vi "SpinnyDebugger.vi"() -> ()   [LabVIEW 2014]
uses:
  <vilib>/userdefined/High Color/IMAQdx.ctl
  <vilib>/LabVIEW Interface for Arduino/LabVIEW Interface for Arduino.lvlib
  <vilib>/vision/driver/NI_Vision_Acquisition_Software.lvlib
  <resource>/objmgr/imaqdx.rc
panel:
  in  "Exposure":u32=3000
  in  "Camera":T1
  out "Image":T2(plugin-control)
  in  "Angular Increment":dbl=5.0
  in  "Captured Image Folder":path
  in  "Camera Mode":enum32{"None", "Triggered", "Live"}(radio)
  in  "Direction":bool=TRUE
  in  "Exit":bool
  in  "home":bool
  in  "stop":bool
  in  "MoveToGo":bool
  in  "Move To":sgl min=0 max=360
  in  "MoveForGo":bool
  in  "Move For (+/-360 max)":sgl=360.0 min=0 max=360
  out "Current Position":sgl format="%.2f"
  # "CW"
  # "CCW"
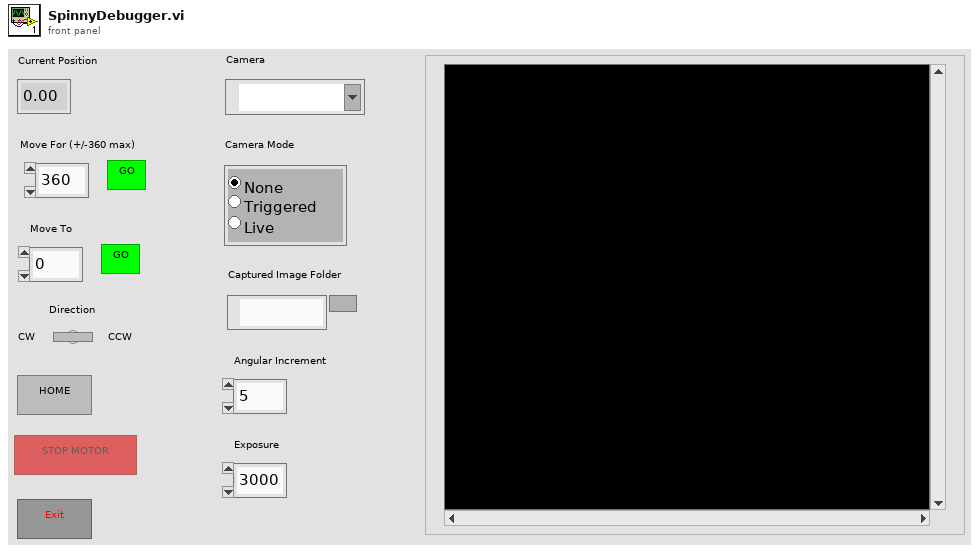
[diagram p1: front panel]
types:
  T1 = typedef "IMAQdx.ctl" = refnum<k21>
  T2 = typedef "IMAQ Image.ctl" = refnum<image>
  T3 = enum8{"Enabled", "Disabled", "Disabled and Grayed Out"}
  T4 = typedef "LabVIEW Interface for Arduino.lvlib/Arduino Resource.ctl" = cluster{"VISA resource":refnum<visa-resource-name>, "Board Type":T5, "Connection Type":enum8{"USB / Serial"}, "Bytes Per Packet (15)":u8}
  T5 = typedef "LabVIEW Interface for Arduino.lvlib/Board Type.ctl" = enum16{"Uno", "Dimuelanove w/Atmega 328", "Mega 2560"}
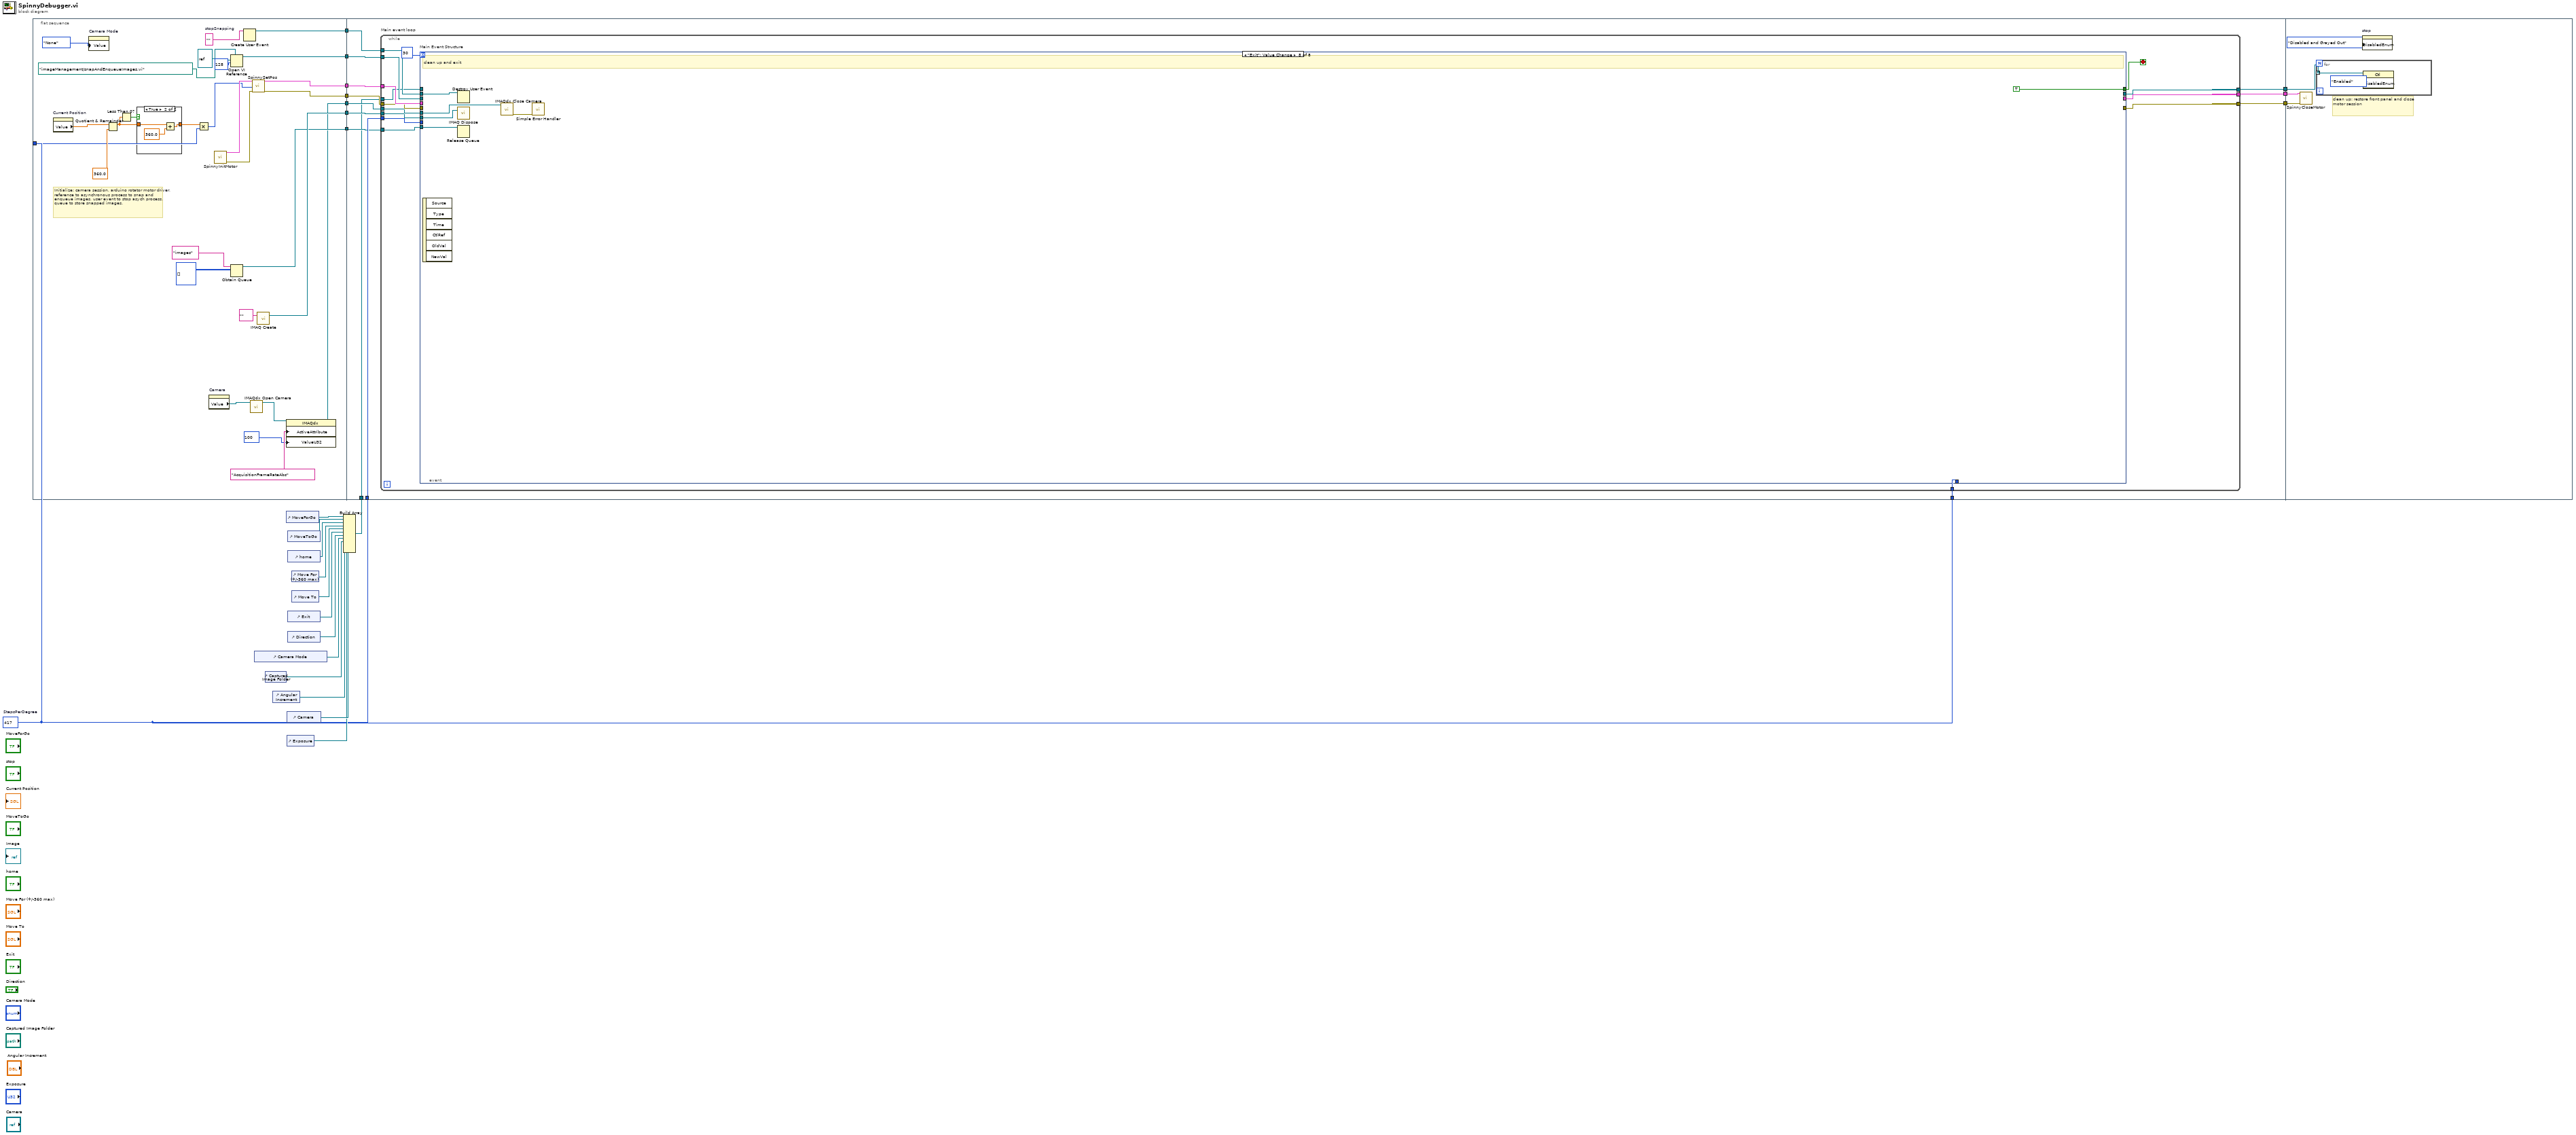
[diagram p0: block diagram]
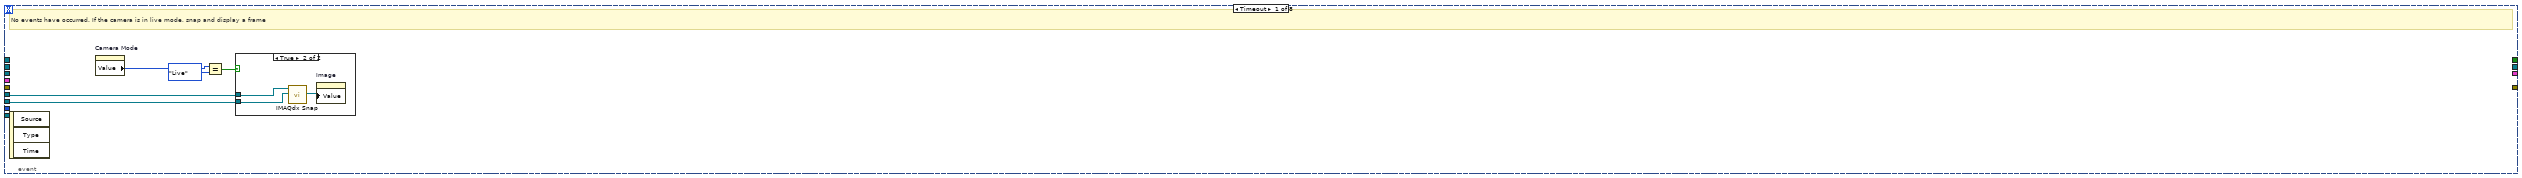
[diagram p3: hidden frame]
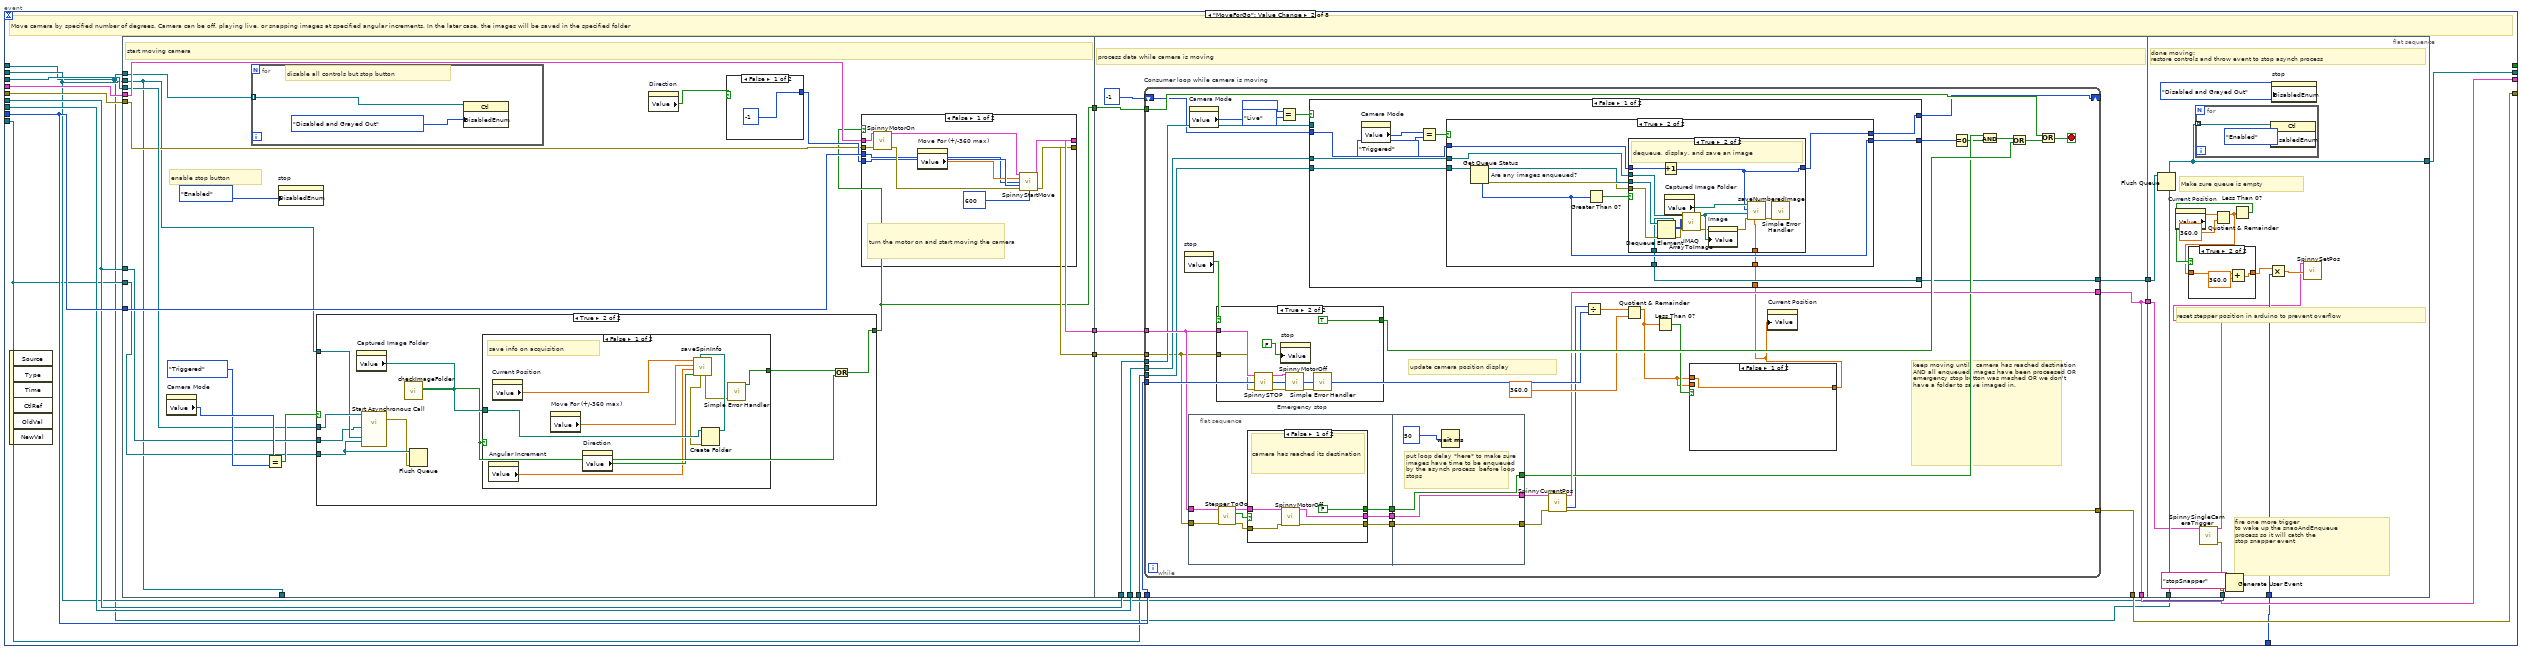
[diagram p5: hidden frame]
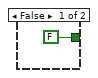
[diagram p7: hidden frame]
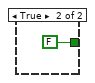
[diagram p8: hidden frame]
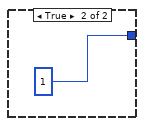
[diagram p9: hidden frame]
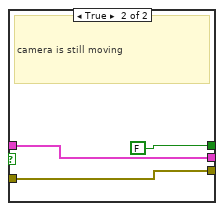
[diagram p10: hidden frame]
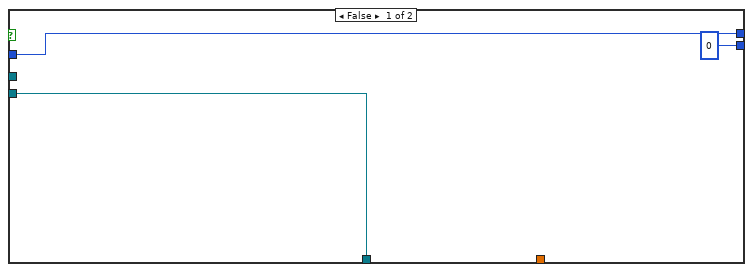
[diagram p11: hidden frame]
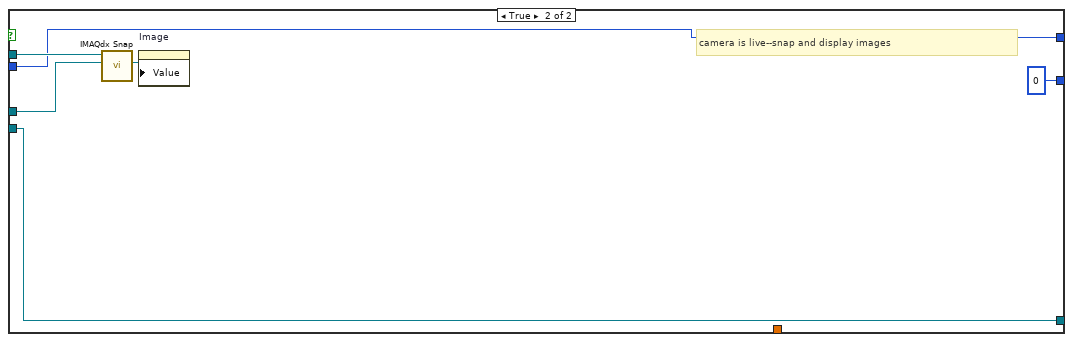
[diagram p13: hidden frame]
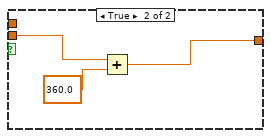
[diagram p14: hidden frame]
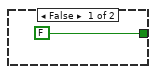
[diagram p15: hidden frame]
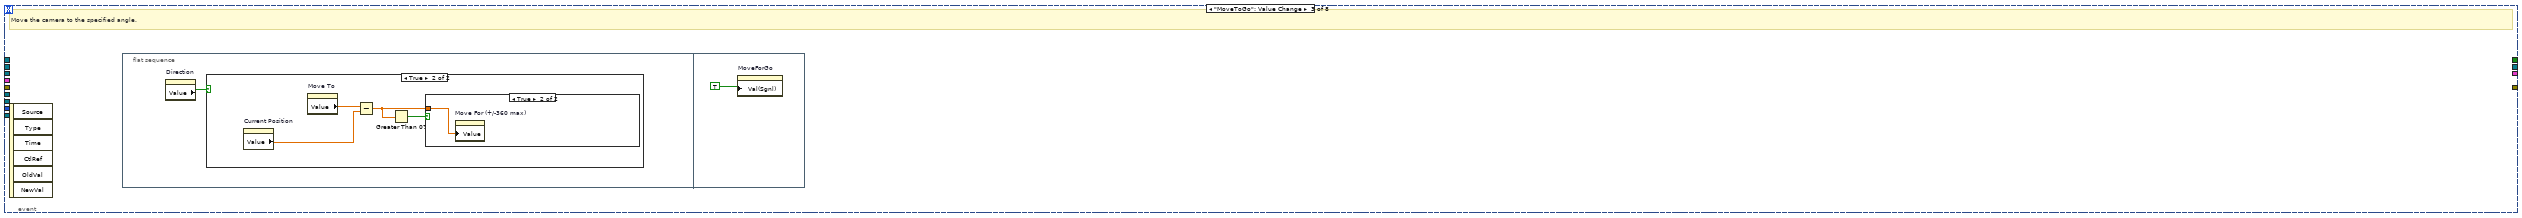
[diagram p17: hidden frame]
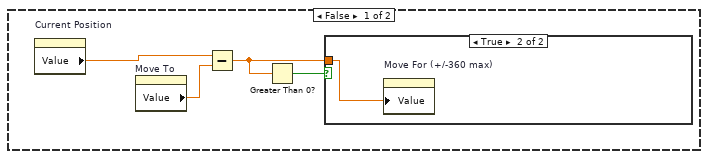
[diagram p18: hidden frame]
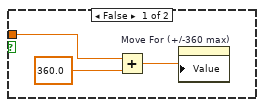
[diagram p19: hidden frame]
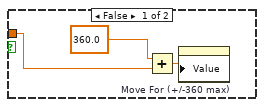
[diagram p20: hidden frame]
diagram:
  w1 = 417  # StepsPerDegree
  n1 = flat-sequence {
    tunnel: [w50] -> w24
    tunnel: [w49] -> w23
    tunnel: w1 -> [w43]
    tunnel: [w27] -> w20
    tunnel: [w39] -> w19
    tunnel: [w33] -> w18
    tunnel: [w31] -> w17
    tunnel: [w30] -> w16
    tunnel: w24 -> [w69]
    tunnel: w23 -> [w68]
    tunnel: w1 -> [w67]
    tunnel: [w66] -> w22
    tunnel: [w65] -> w21
    tunnel: w20 -> [w64]
    tunnel: w19 -> [w63]
    tunnel: w18 -> [w62]
    tunnel: w17 -> [w61]
    tunnel: w16 -> [w60]
    tunnel: w4 -> [w59]
    tunnel: [w58] -> w3
    tunnel: w1 -> [w57]
    tunnel: w22 -> [w384]
    tunnel: w21 -> [w385]
    tunnel: w3 -> [w382]
    frame #0 {
      w32 = ""  # stopSnapping
      # "Initialize: camera session, arduino rotator motor driver, reference to asynchronous process to snap and enqueue images, user event to stop asych process, queue to store snapped images."
      n2 = property on="Current Position" class="DigNum (strict)"() -> ("Value"=w48:sgl)  [unwired: 2 in, 2 out]
      n3 = property on="Camera Mode" class="RadioBtnsControl (strict)"("Value"=enum32{"None", "Triggered"}."None" ("Camera Mode")) -> ()  [unwired: 2 in, 2 out]
      n4 = Quotient & Remainder(x=w48, y=sgl 360.0) -> (x-y*floor(x/y)=w45:sgl)  [unwired: 1 out]
      n5 = Less Than 0?(x=w45) -> (x < 0?=w46:bool)
      n6 = case shown="True" w46 {
        tunnel: w45 -> [w53 w55]
        tunnel: [w53 w54] -> w44
        frame False {
        }
        frame True {
          n7 = Add(x=w55, y=360.0) -> (x+y=w54:dbl)
        }
      }
      n8 = Multiply(x=w44, y=w43) -> (x*y=w42:i32)
      n9 = property on="Camera" class="IMAQdx (strict)"() -> ("Value"=w29:T1)  [unwired: 2 in, 2 out]
      n10 = call "SpinnyInitMotor.vi"() -> ("error out"=w51:errorcluster, "Arduino Resource Out"=w52:T4)  [unwired: 10 in]
      n11 = Open VI Reference(type specifier VI Refnum (for type only)=refnum<vi> refnum, vi path=path "imageManagement/snapAndEnqueueImages.vi", options=128) -> (vi reference=w33:refnum<vi>)  [unwired: 3 in, 1 out]
      n12 = Obtain Queue(name (unnamed)="images", element data type=u8[][] [] ("Image Pixels (U8)")) -> (queue out=w30:refnum<queue>)  [unwired: 3 in, 2 out]
      n13 = Create User Event(user event datatype=w32) -> (user event=w31:refnum<user-event>)  [unwired: 1 in, 1 out]
      n14 = call <vilib>:"IMAQdx Open Camera.vi"("Session In"=w29) -> ("Session Out"=w28:T1)  [unwired: 9 in, 1 out]
      n15 = call "SpinnySetPos.vi"("Arduino Resource"=w52, "position"=w42, "error in"=w51) -> ("Arduino Resource Out"=w50:T4, "error out"=w49:errorcluster)  [unwired: 15 in]
      n16 = call "IMAQ Create"("Image Name"="") -> ("New Image"=w39:T2)  [unwired: 4 in, 1 out]
      n17 = property class="IMAQdx"(reference=w28, "ActiveAttribute"="AcquisitionFrameRateAbs", "ValueU32"=u32 100) -> (reference out=w27:T1)  [unwired: 1 in, 1 out]
    }
    frame #1 {
      n18 = while "Main event loop" {
        tunnel: w69 -> [w83]
        tunnel: w68 -> [w82]
        tunnel: w67 -> [w81]
        tunnel: [w80] -> w66
        tunnel: [w79] -> w65
        tunnel: w64 -> [w77]
        tunnel: w63 -> [w76]
        tunnel: w62 -> [w75]
        tunnel: w61 -> [w74]
        tunnel: w60 -> [w73]
        tunnel: w59 -> [w72]
        tunnel: [w71] -> w58
        tunnel: w57 -> [w70]
        stop <- w84 stop-if-true
        n19 = event "Main Event Structure" shown="[7] \"Exit\": Value Change" {
          selector: _ -> [_ _ _ _ _ _ _ _]
          dyn-events: _ -> [_ _ _ _ _ _ _ _]
          timeout: 30 -> [_ _ _ _ _ _ _ _]
          tunnel: [_ _ _ _ _ _ _ TRUE] -> w84
          tunnel: w83 -> [_ w110 _ w330 _ _ w375 _]
          tunnel: w82 -> [_ w109 _ w329 _ w366 w374 _]
          tunnel: w81 -> [_ w106 _ w328 _ _ _ _]
          tunnel: [_ w105 _ w327 _ _ w372 _] -> w80
          tunnel: [_ w104 _ w326 _ w365 w371 _] -> w79
          tunnel: w77 -> [w89 w102 _ w325 _ w369 _ w381]
          tunnel: w76 -> [w88 w103 _ _ _ _ _ w380]
          tunnel: w75 -> [_ w101 _ _ _ _ _ _]
          tunnel: w74 -> [_ w98 _ _ _ _ _ w378]
          tunnel: w73 -> [_ w97 _ _ _ _ _ w379]
          tunnel: w72 -> [_ w96 _ _ _ _ _ _]
          tunnel: [_ w100 _ _ _ _ _ _] -> w71
          tunnel: w70 -> [_ w94 _ _ _ _ _ _]
          event Timeout {
            # "No events have occurred. If the camera is in live mode, snap and display a frame"
            n20 = event-data() -> ()  [unwired: 1 in, 3 out]
            n21 = property on="Camera Mode" class="RadioBtnsControl (strict)"() -> ("Value"=w87:enum32{"None", "Triggered", "Live"})  [unwired: 2 in, 2 out]
            n22 = Equal?(x=w87, y=enum32{"None", "Triggered", "Live"}."Live") -> (x = y?=w85:bool)
            n23 = case shown="True" w85 {
              tunnel: w89 -> [_ w92]
              tunnel: w88 -> [_ w90]
              frame False {
              }
              frame True {
                n24 = call <vilib>:"IMAQdx Snap.vi"("Image In"=w90, "Session In"=w92) -> ("Image Out"=w91:T2)  [unwired: 7 in, 2 out]
                n25 = property on="Image" class="ImageControl"("Value"=w91) -> ()  [unwired: 2 in, 2 out]
              }
            }
          }
          event "MoveForGo": Value Change {
            # "Move camera by specified number of degrees. Camera can be off, playing live, or snapping images at specified angular increments. In the later case, the images will be saved in the specified folder"
            n26 = event-data() -> ()  [unwired: 1 in, 6 out]
            n27 = flat-sequence {
              tunnel: w110 -> [w127]
              tunnel: w109 -> [w114]
              tunnel: w106 -> [w126]
              tunnel: [w124] -> w108
              tunnel: [w123] -> w107
              tunnel: w102 -> [w119]
              tunnel: w101 -> [w117]
              tunnel: w97 -> [w116]
              tunnel: [w111] -> _
              tunnel: w96 -> [w115]
              tunnel: [w113] -> w99
              tunnel: w98 -> [w111]
              tunnel: w108 -> [w172]
              tunnel: w107 -> [w174]
              tunnel: w106 -> [w173]
              tunnel: [w164] -> w105
              tunnel: [w171] -> w104
              tunnel: w102 -> [w170]
              tunnel: w103 -> [w169]
              tunnel: w97 -> [w168]
              tunnel: w99 -> [w167]
              tunnel: [w165] -> w95
              tunnel: [w164] -> w93
              tunnel: w98 -> [w299]
              tunnel: w96 -> [w297]
              tunnel: [w297] -> w100
              tunnel: w95 -> [w296]
              tunnel: w94 -> [w290]
              tunnel: w93 -> [w288]
              frame #0 {
                # "enable stop button"
                # "start moving camera"
                n28 = property on="Camera Mode" class="RadioBtnsControl (strict)"() -> ("Value"=w121:enum32{"None", "Triggered", "Live"})  [unwired: 2 in, 2 out]
                n29 = for {
                  tunnel: w115 -> [w141] mode=indexing
                  # "disable all controls but stop button"
                  n30 = property on="Property Node" class="Ctl"(reference=w141, "DisabledEnum"=T3."Disabled and Grayed Out" ("Disabled")) -> ()  [unwired: 1 in, 2 out]
                }
                n31 = Equal?(x=w121, y=enum32{"None", "Triggered"}."Triggered") -> (x = y?=w118:bool)
                n32 = property on="stop" class="Bool (strict)"("DisabledEnum"=T3."Enabled" ("Disabled")) -> ()  [unwired: 2 in, 2 out]
                n33 = case shown="True" w118 {
                  tunnel: w119 -> [_ w149]
                  tunnel: w117 -> [_ w151]
                  tunnel: w116 -> [_ w144]
                  tunnel: w111 -> [_ w150]
                  tunnel: [FALSE ("badPath") w145] -> w113
                  frame False {
                  }
                  frame True {
                    n34 = property on="Captured Image Folder" class="Path"() -> ("Value"=w148:path)  [unwired: 2 in, 2 out]
                    n35 = call-by-ref "Start Asynchronous Call"(reference=w151, "queue in"=w144, "user event in"=w150, "Session In"=w149) -> (error out=w143:errorcluster)  [unwired: 10 in, 1 out]
                    n36 = call "checkImageFolder.vi"("Path"=w148) -> ("badPath"=w147:bool)  [unwired: 10 in]
                    n37 = Flush Queue(queue=w144, error in (no error)=w143) -> ()  [unwired: 3 out]
                    n38 = case shown="False" w147 {
                      tunnel: w148 -> [w160 _]
                      tunnel: [w157 FALSE] -> w146
                      frame False {
                        # "save info on acquisition"
                        n39 = property on="Angular Increment" class="DigNum (strict)"() -> ("Value"=w152:dbl)  [unwired: 2 in, 2 out]
                        n40 = property on="Current Position" class="DigNum (strict)"() -> ("Value"=w154:sgl)  [unwired: 2 in, 2 out]
                        n41 = property on="Move For (+/-360 max)" class="DigNum (strict)"() -> ("Value"=w153:sgl)  [unwired: 2 in, 2 out]
                        n42 = property on="Direction" class="Bool (strict)"() -> ("Value"=w158:bool)  [unwired: 2 in, 2 out]
                        n43 = Create Folder(path (use dialog)=w160) -> (created path=w159:path, error out=w156:errorcluster)  [unwired: 2 in, 1 out]
                        n44 = call "saveSpinInfo.vi"("error in (no error)"=w156, "folder"=w159, "direction"=w158, "increment"=w152, "angleToMove"=w153, "startAngle"=w154) -> ("error out"=w155:errorcluster)  [unwired: 5 in]
                        n45 = call <vilib>:"Simple Error Handler.vi"("error in (no error)"=w155) -> ("error?"=w157:bool)  [unwired: 4 in, 4 out]
                      }
                      frame True {
                      }
                    }
                    n46 = Or(x=w146, y=w147) -> (x .or. y?=w145:bool)
                  }
                }
                n47 = property on="Direction" class="Bool (strict)"() -> ("Value"=w112:bool)  [unwired: 2 in, 2 out]
                n48 = case shown="False" w112 {
                  tunnel: [-1 1] -> w122
                  frame False {
                  }
                  frame True {
                  }
                }
                n49 = case shown="False" w113 {
                  tunnel: w127 -> [w137 w138]
                  tunnel: w126 -> [w129 _]
                  tunnel: [w134 w138] -> w124
                  tunnel: [w133 w139] -> w123
                  tunnel: w122 -> [w132 _]
                  tunnel: w114 -> [w130 w139]
                  frame False {
                    # "turn the motor on and start moving the camera"
                    n50 = call "SpinnyMotorOn.vi"("Arduino Resource"=w137, "error in"=w130) -> ("Arduino Resource Out"=w136:T4, "error out"=w135:errorcluster)  [unwired: 12 in]
                    n51 = property on="Move For (+/-360 max)" class="DigNum (strict)"() -> ("Value"=w131:sgl)  [unwired: 2 in, 2 out]
                    n52 = call "SpinnyStartMove.vi"("Arduino Resource"=w136, "Degrees To Move"=w131, "Steps Per Degree"=w129, "Direction"=w132, "error in"=w135, "Max Speed (steps/s)"=u16 600) -> ("Arduino Resource Out"=w134:T4, "error out"=w133:errorcluster)  [unwired: 8 in]
                  }
                  frame True {
                  }
                }
              }
              frame #1 {
                # "process data while camera is moving"
                n53 = while "Consumer loop while camera is moving" {
                  tunnel: w174 -> [w185]
                  tunnel: w173 -> [w207]
                  tunnel: w172 -> [w202]
                  tunnel: [w199] -> w164
                  tunnel: [w198] -> w171
                  tunnel: w170 -> [w194]
                  tunnel: w169 -> [w193]
                  tunnel: w168 -> [w192]
                  tunnel: w167 -> [w189]
                  shift-right: [w186] -> _
                  shift-left: -1 -> [w187]
                  tunnel: [w176] -> w165
                  stop <- w188 stop-if-true
                  # "keep moving untill  camera has reached destination AND all enqueued images have been proceesed OR emergency stop button was mashed OR we don't have a folder to save imaged in."
                  # "update camera position display"
                  n54 = property on="stop" class="Bool (strict)"() -> ("Value"=w191:bool)  [unwired: 2 in, 2 out]
                  n55 = flat-sequence {
                    tunnel: w202 -> [w213]
                    tunnel: w185 -> [w210]
                    tunnel: [w212] -> w180
                    tunnel: [w211] -> w179
                    tunnel: [w209] -> w178
                    tunnel: [w226] -> w182
                    tunnel: [w227] -> w200
                    tunnel: [w228] -> w201
                    tunnel: w180 -> [w228]
                    tunnel: w179 -> [w227]
                    tunnel: w178 -> [w226]
                    frame #0 {
                      n56 = call <vilib>:"Stepper ToGo.vi"("error in"=w210, "Arduino Resource"=w213) -> ("error out"=w214:errorcluster, "Steps Remaining?"=w216:bool, "Arduino Resource Out"=w215:T4)  [unwired: 6 in, 1 out]
                      n57 = case shown="False" w216 {
                        tunnel: w215 -> [w221 w222]
                        tunnel: w214 -> [w220 w223]
                        tunnel: [FALSE FALSE] -> w209
                        tunnel: [w218 w222] -> w212
                        tunnel: [w217 w223] -> w211
                        frame False {
                          # "camera has reached its destination"
                          n58 = call "SpinnyMotorOff.vi"("Arduino Resource"=w221, "error in"=w220) -> ("Arduino Resource Out"=w218:T4, "error out"=w217:errorcluster)  [unwired: 12 in]
                        }
                        frame True {
                          # "camera is still moving"
                        }
                      }
                    }
                    frame #1 {
                      # "put loop delay *here* to make sure images have time to be enqueued by the asynch process  before loop stops"
                      n59 = Wait (ms)(milliseconds to wait=u32 50) -> ()  [unwired: 1 out]
                    }
                  }
                  n60 = property on="Camera Mode" class="RadioBtnsControl (strict)"() -> ("Value"=w197:enum32{"None", "Triggered", "Live"})  [unwired: 2 in, 2 out]
                  n61 = case "Emergency stop" shown="True" w191 {
                    tunnel: [FALSE TRUE] -> w208
                    tunnel: w202 -> [_ w282]
                    tunnel: w185 -> [_ w281]
                    frame False {
                    }
                    frame True {
                      n62 = call "SpinnySTOP.vi"("error in"=w281, "Arduino Resource"=w282) -> ("error out"=w283:errorcluster, "Arduino Resource Out"=w284:T4)  [unwired: 8 in]
                      n63 = property on="stop" class="Bool (strict)"("Value"=FALSE ("stop")) -> ()  [unwired: 2 in, 2 out]
                      n64 = call "SpinnyMotorOff.vi"("Arduino Resource"=w284, "error in"=w283) -> ("error out"=w279:errorcluster)  [unwired: 12 in, 1 out]
                      n65 = call <vilib>:"Simple Error Handler.vi"("error in (no error)"=w279) -> ()  [unwired: 4 in, 5 out]
                    }
                  }
                  n66 = Equal?(x=w197, y=enum32{"None", "Triggered", "Live"}."Live") -> (x = y?=w195:bool)
                  n67 = call "SpinnyCurrentPos.vi"("Arduino Resource"=w201, "error in"=w200) -> ("Arduino Resource Out"=w199:T4, "position"=w177:i32, "error out"=w198:errorcluster)  [unwired: 15 in]
                  n68 = Divide(x=w177, y=w207) -> (x/y=w206:sgl)
                  n69 = Quotient & Remainder(x=w206, y=sgl 360.0) -> (x-y*floor(x/y)=w203:sgl)  [unwired: 1 out]
                  n70 = Less Than 0?(x=w203) -> (x < 0?=w204:bool)
                  n71 = case shown="False" w204 {
                    tunnel: w203 -> [_ w277]
                    tunnel: [w274 w275] -> w175
                    tunnel: w203 -> [w274 _]
                    frame False {
                    }
                    frame True {
                      n72 = Add(x=w277, y=sgl 360.0) -> (x+y=w275:sgl)
                    }
                  }
                  n73 = case shown="False" w195 {
                    tunnel: w194 -> [_ w273]
                    tunnel: w193 -> [w234 w272]
                    tunnel: w192 -> [w235 w268]
                    tunnel: w187 -> [w233 w270]
                    tunnel: [w232 w270] -> w186
                    tunnel: [w231 0 ("# elements in queue")] -> w184
                    tunnel: [w230 w268] -> w176
                    tunnel: w175 -> [w229 _]
                    frame False {
                      n74 = property on="Camera Mode" class="RadioBtnsControl (strict)"() -> ("Value"=w238:enum32{"None", "Triggered", "Live"})  [unwired: 2 in, 2 out]
                      n75 = Equal?(x=w238, y=enum32{"None", "Triggered", "Live"}."Triggered") -> (x = y?=w236:bool)
                      n76 = case shown="True" w236 {
                        tunnel: w235 -> [w239 w251]
                        tunnel: w234 -> [_ w248]
                        tunnel: w233 -> [w241 w247]
                        tunnel: [w241 w244] -> w232
                        tunnel: [0 ("# elements in queue") w245] -> w231
                        tunnel: [w239 w243] -> w230
                        tunnel: w229 -> [_ w242]
                        frame False {
                        }
                        frame True {
                          n77 = Get Queue Status "Are any images enqueued?"(queue=w251) -> (queue out=w249:refnum<queue>, error out=w246:errorcluster, # elements in queue=w245:i32)  [unwired: 2 in, 5 out]
                          n78 = Greater Than 0?(x=w245) -> (x > 0?=w250:bool)
                          n79 = case shown="True" w250 {
                            tunnel: w249 -> [w252 w267]
                            tunnel: w248 -> [_ w265]
                            tunnel: w247 -> [w253 w257]
                            tunnel: [w253 w256] -> w244
                            tunnel: w246 -> [_ w262]
                            tunnel: [w252 w255] -> w243
                            tunnel: w242 -> [_ w254]
                            frame False {
                            }
                            frame True {
                              # "dequeue, display, and save an image"
                              n80 = Dequeue Element(queue=w267, error in (no error)=w262) -> (queue out=w255:refnum<queue>, element=w266:u8[][], error out=w261:errorcluster)  [unwired: 1 in, 1 out]
                              n81 = Increment(x=w257) -> (x+1=w256:i32)
                              n82 = property on="Captured Image Folder" class="Path"() -> ("Value"=w263:path)  [unwired: 2 in, 2 out]
                              n83 = call "IMAQ ArrayToImage"("error in (no error)"=w261, "Image Pixels (U8)"=w266, "Image"=w265) -> ("error out"=w260:errorcluster, "Image Out"=w264:T2)  [unwired: 7 in]
                              n84 = property on="Image" class="ImageControl"(error in=w260, "Value"=w264) -> (error out=w258:errorcluster)  [unwired: 1 in, 1 out]
                              n85 = call "saveNumberedImage.vi"("currentPos"=w254, "error in (no error)"=w258, "Image"=w264, "imageNumber"=w256, "folder"=w263) -> ("error out"=w259:errorcluster)  [unwired: 6 in]
                              n86 = call <vilib>:"Simple Error Handler.vi"("error in (no error)"=w259) -> ()  [unwired: 4 in, 5 out]
                            }
                          }
                        }
                      }
                    }
                    frame True {
                      # "camera is live--snap and display images"
                      n87 = call <vilib>:"IMAQdx Snap.vi"("Image In"=w272, "Session In"=w273) -> ("Image Out"=w271:T2)  [unwired: 7 in, 2 out]
                      n88 = property on="Image" class="ImageControl"("Value"=w271) -> ()  [unwired: 2 in, 2 out]
                    }
                  }
                  n89 = property on="Current Position" class="DigNum (strict)"("Value"=w175) -> ()  [unwired: 2 in, 2 out]
                  n90 = Equal To 0?(x=w184) -> (x = 0?=w181:bool)
                  n91 = And(x=w182, y=w181) -> (x .and. y?=w183:bool)
                  n92 = Or(x=w183, y=w208) -> (x .or. y?=w190:bool)
                  n93 = Or(x=w189, y=w190) -> (x .or. y?=w188:bool)
                }
              }
              frame #2 {
                # "fire one more trigger \nto wake up the snaoAndEnqueue\nprocess so it will catch the \nstop snapper event"
                # "reset stepper position in arduino to prevent overflow"
                # "Make sure queue is empty"
                # "done moving: \nrestore controls and throw event to stop asynch process"
                n94 = Flush Queue(queue=w296) -> ()  [unwired: 1 in, 3 out]
                n95 = property on="Current Position" class="DigNum (strict)"() -> ("Value"=w295:sgl)  [unwired: 2 in, 2 out]
                n96 = for {
                  tunnel: w297 -> [w306] mode=indexing
                  n97 = property class="Ctl"(reference=w306, "DisabledEnum"=T3."Enabled" ("Disabled")) -> ()  [unwired: 1 in, 2 out]
                }
                n98 = call "SpinnySingleCameraTrigger.vi"("Arduino Resource"=w288) -> ("error out"=w286:errorcluster, "Arduino Resource Out"=w287:T4)  [unwired: 9 in]
                n99 = Quotient & Remainder(x=w295, y=sgl 360.0) -> (x-y*floor(x/y)=w292:sgl)  [unwired: 1 out]
                n100 = Generate User Event(user event=w299, event data cluster="stopSnapper", error in=w286) -> ()  [unwired: 1 in, 2 out]
                n101 = Less Than 0?(x=w292) -> (x < 0?=w293:bool)
                n102 = case shown="True" w293 {
                  tunnel: w292 -> [w301 w303]
                  tunnel: [w301 w302] -> w291
                  frame False {
                  }
                  frame True {
                    n103 = Add(x=w303, y=360.0) -> (x+y=w302:dbl)
                  }
                }
                n104 = Multiply(x=w291, y=w290) -> (x*y=w289:dbl)
                n105 = property on="stop" class="Bool (strict)"("DisabledEnum"=T3."Disabled and Grayed Out" ("Disabled")) -> ()  [unwired: 2 in, 2 out]
                n106 = call "SpinnySetPos.vi"("Arduino Resource"=w287, "position"=w289) -> ()  [unwired: 16 in, 2 out]
              }
            }
          }
          event "MoveToGo": Value Change {
            # "Move the camera to the specified angle."
            n107 = event-data() -> ()  [unwired: 1 in, 6 out]
            n108 = flat-sequence {
              frame #0 {
                n109 = property on="Direction" class="Bool (strict)"() -> ("Value"=w307:bool)  [unwired: 2 in, 2 out]
                n110 = case shown="True" w307 {
                  frame False {
                    n111 = property on="Current Position" class="DigNum (strict)"() -> ("Value"=w311:sgl)  [unwired: 2 in, 2 out]
                    n112 = property on="Move To" class="DigNum (strict)"() -> ("Value"=w310:sgl)  [unwired: 2 in, 2 out]
                    n113 = Subtract(x=w311, y=w310) -> (x-y=w308:sgl)
                    n114 = Greater Than 0?(x=w308) -> (x > 0?=w309:bool)
                    n115 = case shown="True" w309 {
                      tunnel: w308 -> [w313 w315]
                      frame False {
                        n116 = Add(x=w313, y=sgl 360.0) -> (x+y=w314:sgl)
                        n117 = property on="Move For (+/-360 max)" class="DigNum (strict)"("Value"=w314) -> ()  [unwired: 2 in, 2 out]
                      }
                      frame True {
                        n118 = property on="Move For (+/-360 max)" class="DigNum (strict)"("Value"=w315) -> ()  [unwired: 2 in, 2 out]
                      }
                    }
                  }
                  frame True {
                    n119 = property on="Current Position" class="DigNum (strict)"() -> ("Value"=w317:sgl)  [unwired: 2 in, 2 out]
                    n120 = property on="Move To" class="DigNum (strict)"() -> ("Value"=w316:sgl)  [unwired: 2 in, 2 out]
                    n121 = Subtract(x=w316, y=w317) -> (x-y=w318:sgl)
                    n122 = Greater Than 0?(x=w318) -> (x > 0?=w319:bool)
                    n123 = case shown="True" w319 {
                      tunnel: w318 -> [w322 w323]
                      frame False {
                        n124 = Add(x=360.0, y=w322) -> (x+y=w321:dbl)
                        n125 = property on="Move For (+/-360 max)" class="DigNum (strict)"("Value"=w321) -> ()  [unwired: 2 in, 2 out]
                      }
                      frame True {
                        n126 = property on="Move For (+/-360 max)" class="DigNum (strict)"("Value"=w323) -> ()  [unwired: 2 in, 2 out]
                      }
                    }
                  }
                }
              }
              frame #1 {
                n127 = property on="MoveForGo" class="Bool (strict)"("Val(Sgnl)"=TRUE ("Value (Signaling)")) -> ()  [unwired: 2 in, 2 out]
              }
            }
          }
          event "Camera Mode": Value Change {
            n128 = event-data() -> ()  [unwired: 1 in, 6 out]
            n129 = property on="Camera Mode" class="RadioBtnsControl (strict)"() -> ("Value"=w332:enum32{"None", "Triggered", "Live"})  [unwired: 2 in, 2 out]
            n130 = Equal?(x=w332, y=enum32{"None", "Live", "Triggered"}."None") -> (x = y?=w333:bool)
            n131 = case shown="False" w333 {
              tunnel: w332 -> [_ _]
              tunnel: w330 -> [w342 w362]
              tunnel: w329 -> [w335 w363]
              tunnel: w328 -> [w341 _]
              tunnel: [w340 w362] -> w327
              tunnel: [w339 w363] -> w326
              tunnel: w325 -> [w334 w359]
              frame False {
                n132 = property on="Camera Mode" class="RadioBtnsControl (strict)"() -> ("Value"=w338:enum32{"None", "Triggered", "Live"})  [unwired: 2 in, 2 out]
                n133 = Equal?(x=w338, y=enum32{"None", "Triggered", "Live"}."Triggered") -> (x = y?=w336:bool)
                n134 = case shown="False" w336 {
                  tunnel: w342 -> [w346 w358]
                  tunnel: w341 -> [_ w357]
                  tunnel: [w346 w355] -> w340
                  tunnel: [w347 w354] -> w339
                  tunnel: w335 -> [w347 w349]
                  tunnel: w334 -> [w345 w351]
                  frame False {
                    # "turn off trigger mode"
                    n135 = property class="IMAQdx"(reference=w345, "ActiveAttribute"="TriggerMode", "ValueU32"=u32 0) -> ()  [unwired: 1 in, 2 out]
                  }
                  frame True {
                    # "turn on trigger mode and tell arduino how often to issue camer tigger signal"
                    n136 = property on="Angular Increment" class="DigNum (strict)"() -> ("Value"=w350:dbl)  [unwired: 2 in, 2 out]
                    n137 = property class="IMAQdx"(reference=w351, error in=w349, "ActiveAttribute"="TriggerMode", "ValueU32"=u32 1) -> (error out=w348:errorcluster)  [unwired: 1 out]
                    n138 = Multiply(x=w350, y=w357) -> (x*y=w356:u16)
                    n139 = call "SpinnyConfigCameraTrigger.vi"("error in"=w348, "triggerInterval"=w356, "Arduino Resource"=w358) -> ("error out"=w354:errorcluster, "Arduino Resource Out"=w355:T4)  [unwired: 7 in]
                  }
                }
              }
              frame True {
                # "turn off trigger mode"
                n140 = property class="IMAQdx"(reference=w359, "ActiveAttribute"="TriggerMode", "ValueU32"=u32 0) -> ()  [unwired: 1 in, 2 out]
              }
            }
          }
          event "Angular Increment": Value Change {
            n141 = event-data() -> ()  [unwired: 1 in, 6 out]
            n142 = property on="Camera Mode" class="RadioBtnsControl (strict)"() -> ("Value"=w364:enum32{"None", "Triggered", "Live"})  [unwired: 2 in, 2 out]
            n143 = property on="Camera Mode" class="RadioBtnsControl (strict)"("Val(Sgnl)"=w364) -> ()  [unwired: 2 in, 2 out]
          }
          event "Exposure": Value Change {
            n144 = event-data() -> ()  [unwired: 1 in, 6 out]
            n145 = property on="Exposure" class="DigNum (strict)"() -> ("Value"=w367:u32)  [unwired: 2 in, 2 out]
            n146 = property class="IMAQdx"(reference=w369, error in=w366, "ActiveAttribute"="ExposureTimeAbs", "ValueU32"=w367) -> (error out=w365:errorcluster)  [unwired: 1 out]
          }
          event "home": Value Change {
            n147 = event-data() -> ()  [unwired: 1 in, 6 out]
            n148 = property on="Current Position" class="DigNum (strict)"("Value"=sgl 0.0 ("Current Position")) -> ()  [unwired: 2 in, 2 out]
            n149 = call "SpinnySetPos.vi"("Arduino Resource"=w375, "position"=i16 0, "error in"=w374) -> ("Arduino Resource Out"=w372:T4, "error out"=w371:errorcluster)  [unwired: 15 in]
          }
          event "Exit": Value Change {
            # "clean up and exit"
            n150 = event-data() -> ()  [unwired: 1 in, 6 out]
            n151 = Destroy User Event(user event=w378) -> ()  [unwired: 1 in, 1 out]
            n152 = call "IMAQ Dispose"("Image"=w380) -> ()  [unwired: 5 in, 1 out]
            n153 = Release Queue(queue=w379) -> ()  [unwired: 2 in, 3 out]
            n154 = call <vilib>:"IMAQdx Close Camera.vi"("Session In"=w381) -> ("error out"=w376:errorcluster)  [unwired: 10 in]
            n155 = call <vilib>:"Simple Error Handler.vi"("error in (no error)"=w376) -> ()  [unwired: 4 in, 5 out]
          }
        }
      }
    }
    frame #2 {
      # "clean up: restore front panel and close motor session"
      n156 = call "SpinnyCloseMotor.vi"("Arduino Resource"=w384, "error in"=w385) -> ()  [unwired: 18 in]
      n157 = for {
        tunnel: w382 -> [w386] mode=indexing
        n158 = property class="Ctl"(reference=w386, "DisabledEnum"=T3."Enabled" ("Disabled")) -> ()  [unwired: 1 in, 2 out]
      }
      n159 = property on="stop" class="Bool (strict)"("DisabledEnum"=T3."Disabled and Grayed Out" ("Disabled")) -> ()  [unwired: 2 in, 2 out]
    }
  }
  n160 = control-ref of="Camera Mode"() -> (w8:refnum<vi>)
  n161 = control-ref of="Captured Image Folder"() -> (w7:refnum<vi>)
  n162 = control-ref of="Angular Increment"() -> (w6:refnum<vi>)
  n163 = control-ref of="MoveForGo"() -> (w15:refnum<vi>)
  n164 = control-ref of="Exposure"() -> (w2:refnum<vi>)
  n165 = control-ref of="Camera"() -> (w5:refnum<vi>)
  n166 = control-ref of="MoveToGo"() -> (w14:refnum<vi>)
  n167 = control-ref of="home"() -> (w13:refnum<vi>)
  n168 = control-ref of="Exit"() -> (w10:refnum<vi>)
  n169 = control-ref of="Direction"() -> (w9:refnum<vi>)
  n170 = control-ref of="Move For (+/-360 max)"() -> (w12:refnum<vi>)
  n171 = control-ref of="Move To"() -> (w11:refnum<vi>)
  n172 = Build Array(w15, w14, w13, w12, w11, w10, w9, w8, w7, w6, w5, w2) -> (w4:refnum<vi>[])
